vi "SEA_9811_Write.vi"(8 "error in (no error)":errorcluster, 10 "Tx Data":T1 format="%032b", 11 "SEA9811_RT_data in":T2 {"Tx"."Tx Refs (Data,Trig)"."Data Reference" format="%.0x"}) -> (0 "error out":errorcluster, 3 "SEA9811_RT_data out":T2 {"Tx"."Tx Refs (Data,Trig)"."Data Reference" format="%.0x"})   [LabVIEW 2012]
doc: "transmit one word immediately"
uses:
  Typdefs/SEA9811_RT_data_cluster.ctl
  <userlib>/_FPGA Interface Advanced Tools/FPGA Interface Base/FPGA Interface Base.lvclass
  Typdefs/FPGA ref.ctl
  Typdefs/channel.ctl
  Typdefs/received word.ctl
  Typdefs/SEA9811_FPGA_FP_Addresses.ctl
  <vilib>/NI Veristand/Custom Device API/Block Data Reference.ctl
  <vilib>/NI Veristand/Custom Device API/Data Reference.ctl
  Typdefs/ARINC word.ctl
  <vilib>/Utility/error.llb/Error Cluster From Error Code.vi
  <vilib>/rvi/errors/niLvFpgaAdjustHostInterfaceError.vi
  <vilib>/rvi/interface/nirviReadWriteControl/nirviReadWriteControl.xnode
  FPGA Bitfiles/SEA-9811_FPGA_9082__9862_9862_9811_9220.lvbitx
  NiFpgaLv.dll
  <vilib>/NI Veristand/Custom Device API/Custom Device API.lvlib
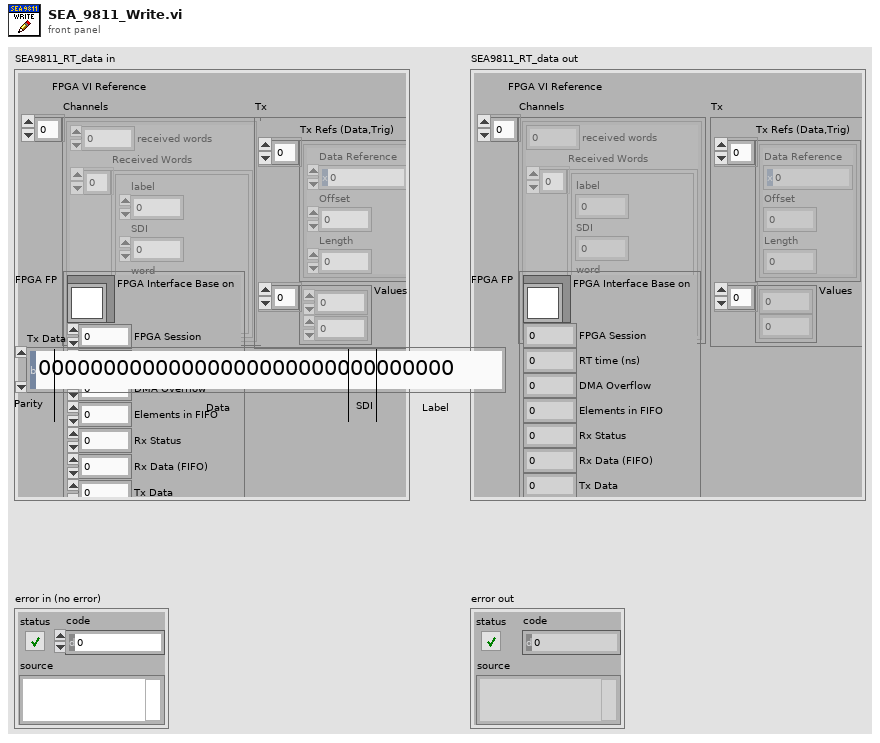
[diagram p1: front panel]
types:
  T1 = typedef "ARINC word.ctl" = u32
  T2 = typedef "SEA9811_RT_data_cluster.ctl" = cluster{"FPGA VI Reference":T3, "Channels":T4[], "FPGA FP":T6, "Tx":cluster{"Tx Refs (Data,Trig)":T7[], "Values":dbl[]}}
  T3 = typedef "FPGA ref.ctl" = refnum<k20>
  T4 = typedef "channel.ctl" = cluster{"received words":u32, "Received Words":T5[]}
  T5 = typedef "received word.ctl" = cluster{"label":u8, "SDI":u8, "word":u32, "timestamp":dbl}
  T6 = typedef "SEA9811_FPGA_FP_Addresses.ctl" = cluster{"FPGA Interface Base on":refnum<class "FPGA Interface Base.lvclass">, "FPGA Session":u32, "RT time (ns)":u32, "DMA Overflow":u32, "Elements in FIFO":u32, "Rx Status":u32, "Rx Data (FIFO)":u32, "Tx Data":u32, "Transmit Data":u32}
  T7 = typedef "Custom Device API.lvlib/Block Data Reference.ctl" = cluster{"Data Reference":T8, "Offset":i32, "Length":i32}
  T8 = typedef "Custom Device API.lvlib/Data Reference.ctl" = i32
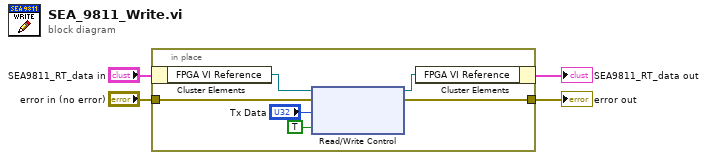
[diagram p0: block diagram]
diagram:
  n1 = in-place {
    in-place-border: "error in (no error)" -> [w9]
    in-place-border: [w8] -> w3
    n2 = in-place-cluster #1("SEA9811_RT_data in") -> ("FPGA VI Reference"=w6:T3)
    n3 = xnode "Read/Write Control"("FPGA VI Reference In"=w6, "error in"=w9, "Tx Data"="Tx Data", "Transmit Data"=TRUE) -> ("FPGA VI Reference Out"=w5:T3, "error out"=w8:errorcluster)
    n4 = in-place-cluster #1("FPGA VI Reference"=w5) -> (→"SEA9811_RT_data out":T2)
  }
  "error out" <- w3
